vi "AviTrack2v2points(13_05_24).vi"() -> ()   [LabVIEW 2015]
uses:
  <vilib>/vision/Image Controls.llb/IMAQ Image.ctl
  <vilib>/vision/NI_Vision_Development_Module.lvlib
  <vilib>/ptbypt/NI_PtbyPt.lvlib
panel:
  out "Number of Matches (Color Location 2)":i32
  out "Number of Matches (Color Location 1)":i32
  out "substring":string
  in  "Enable":bool
  out "x+1":i32
  out "decimal integer string":string
  out "error out 2":errorcluster caption="error out"
  out "Saving Data":bool
  in  "error in (no error)":errorcluster
  out "Tiempo 2":dbl
  out "Tiempo":dbl
  out "Waveform Chart":dbl[](graph)
  out "Threshold":T1(plugin-control)
  out "Global Rectangle":dbl[](array[numeric])
  out "1°":i32
  out "2°":i32
  out "Dif. Puntos":i32
  in  "x = Centimetros reales":i32=20
  out "Dif. CM":dbl
  out "Waveform Chart 3":dbl(graph)
  out "Dist. CM":sgl
  out "Dist. Pixel":sgl
  out "IMA 3":T1(plugin-control)
  in  "Blue or Luminance":cluster{i32, i32}(slide)={0, 191} scale=0.0..255.0
  in  "Green or Saturation":cluster{i32, i32}(slide)={40, 231} scale=0.0..255.0
  in  "Red or Hue":cluster{i32, i32}(slide)={86, 222} scale=0.0..255.0
  out "Bounding Box[0].x":sgl
  out "error out":errorcluster
  out "Progress Bar 2":i32(slide) max=25 scale=-1.0..162.0
  in  "base path 2":path
  in  "Color Mode":u16(ring)=1 items=["RGB", "HSL", "HSV", "HSI"]
  out "Image":T1(plugin-control)
  in  "stop":bool
  out "Image Dst Out":T1
  out "Image 2":T1(plugin-control)
  in  "invert":bool
  out "IMA 2":T1(plugin-control)
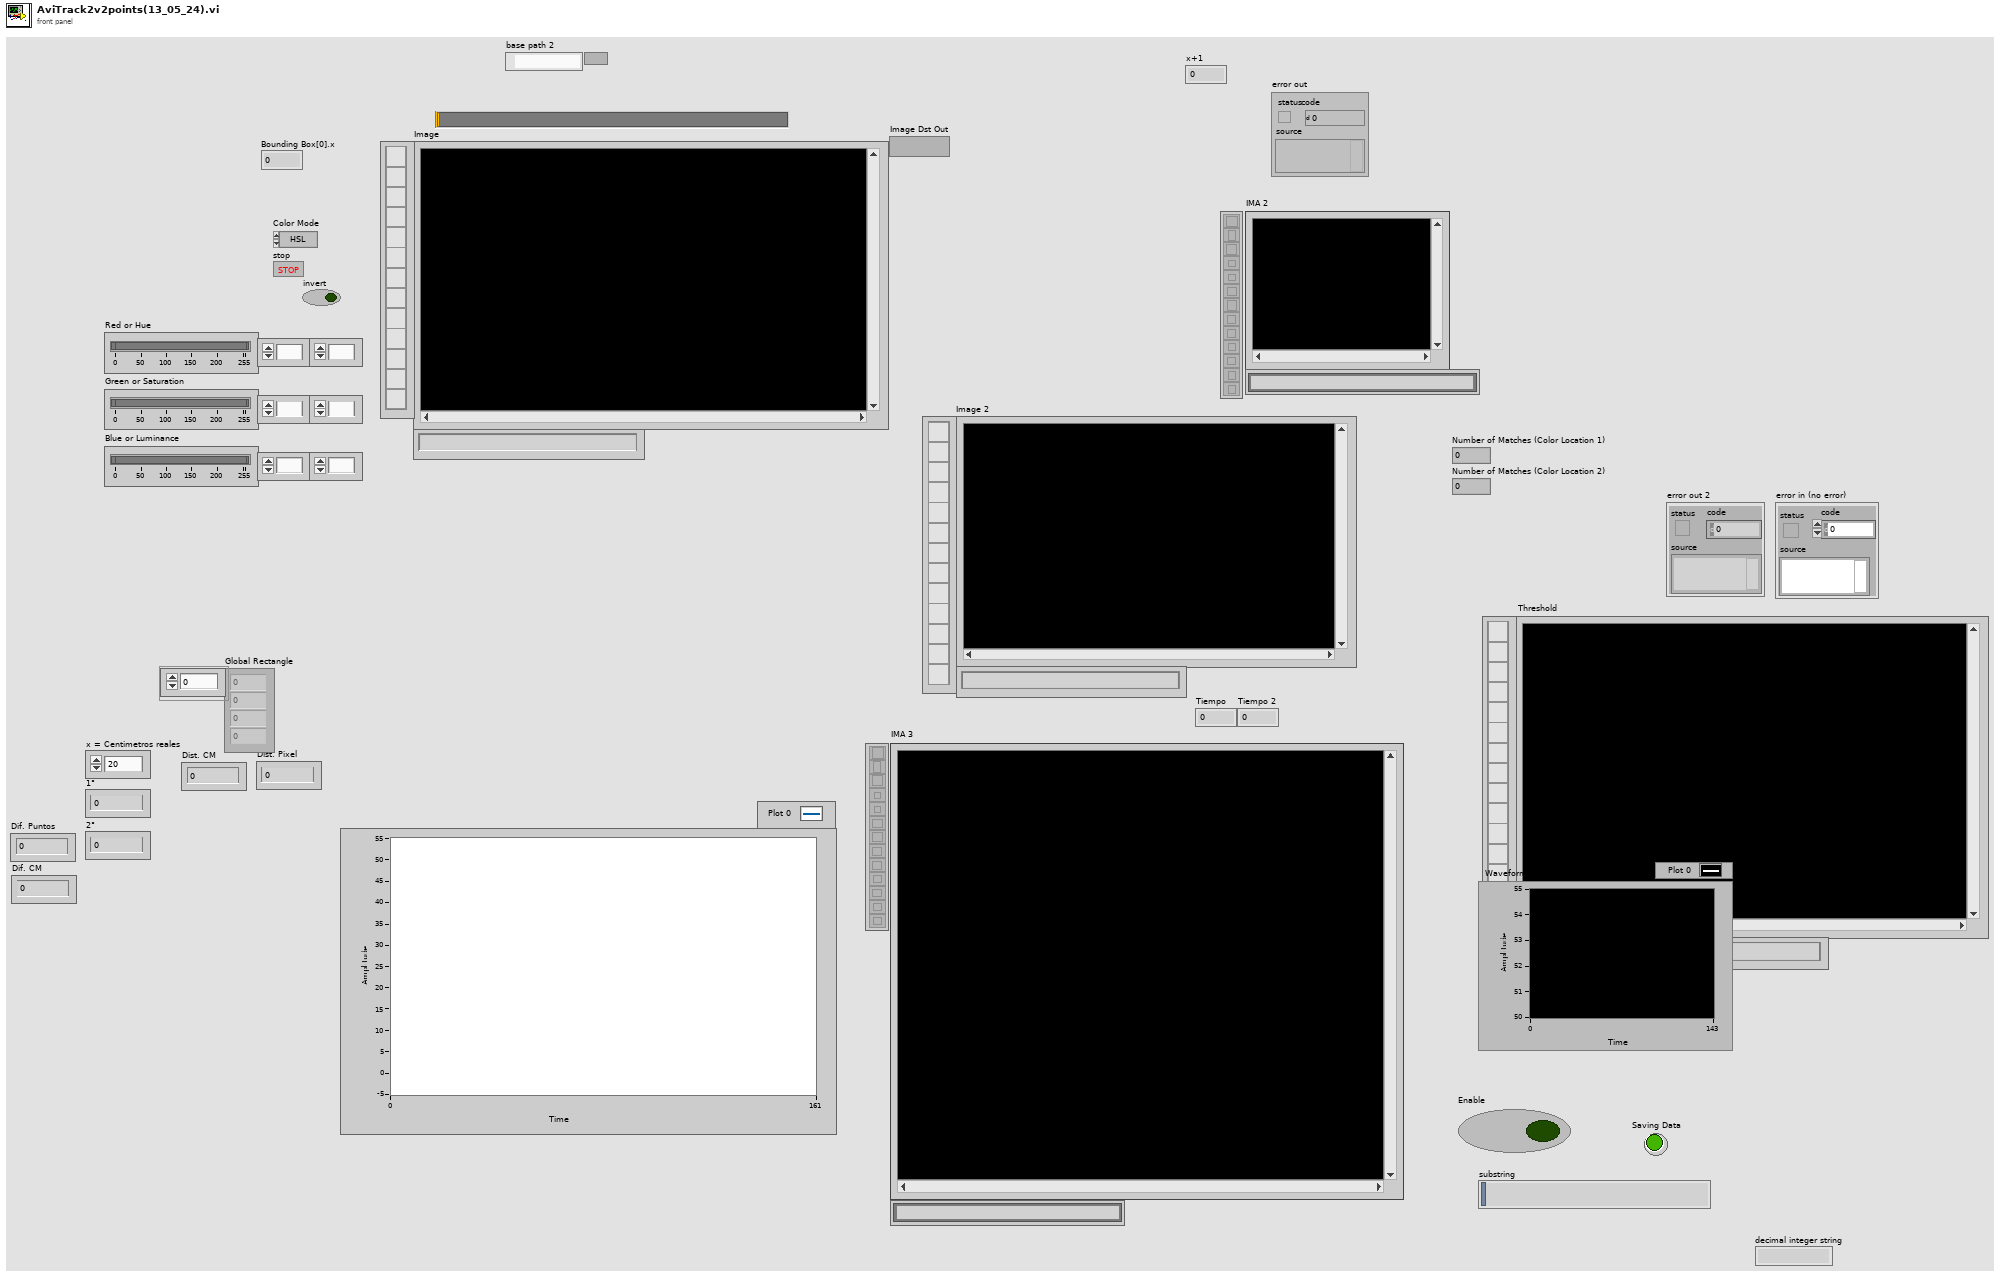
[diagram p1: front panel]
types:
  T1 = typedef "IMAQ Image.ctl" = refnum<image>
  T2 = typedef "Image Type" = u32
  T3 = typedef "IMAQ AVI2 Refnum.ctl" = refnum<k20>
  T4 = cluster{"Width":u32, "Height":u32, "Frames Per Second":u32, "Codec":string, "Has Data":bool}
  T5 = cluster{"Global Rectangle":i32[], "Contours":cluster{"Contour Type":u32, "ROI Type":u32, "Points":i32[]}[]}
  T6 = cluster{"Position":cluster{"x":sgl, "y":sgl}, "Angle":sgl, "Scale":sgl, "Score":sgl, "Bounding Box":cluster{"x":sgl, "y":sgl}[]}[]
  T7 = cluster{"Position":cluster{"x":sgl, "y":sgl}, "Angle":sgl, "Scale":sgl, "Score":sgl, "Bounding Box":cluster{"x":sgl, "y":sgl}[]}
  T8 = cluster{"Matches (Color Location 1)[0]":cluster{"Position":cluster{"x":sgl, "y":sgl}, "Angle":sgl, "Scale":sgl, "Score":sgl, "Bounding Box":cluster{"x":sgl, "y":sgl}[]}, "Matches (Color Location 1)[1]":cluster{"Position":cluster{"x":sgl, "y":sgl}, "Angle":sgl, "Scale":sgl, "Score":sgl, "Bounding Box":cluster{"x":sgl, "y":sgl}[]}, "Matches (Color Location 1)[2]":cluster{"Position":cluster{"x":sgl, "y":sgl}, "Angle":sgl, "Scale":sgl, "Score":sgl, "Bounding Box":cluster{"x":sgl, "y":sgl}[]}, "Matches (Color Location 1)[3]":cluster{"Position":cluster{"x":sgl, "y":sgl}, "Angle":sgl, "Scale":sgl, "Score":sgl, "Bounding Box":cluster{"x":sgl, "y":sgl}[]}}
  T9 = cluster{"Matches (Color Location 2)[0]":cluster{"Position":cluster{"x":sgl, "y":sgl}, "Angle":sgl, "Scale":sgl, "Score":sgl, "Bounding Box":cluster{"x":sgl, "y":sgl}[]}, "Matches (Color Location 2)[1]":cluster{"Position":cluster{"x":sgl, "y":sgl}, "Angle":sgl, "Scale":sgl, "Score":sgl, "Bounding Box":cluster{"x":sgl, "y":sgl}[]}, "Matches (Color Location 2)[2]":cluster{"Position":cluster{"x":sgl, "y":sgl}, "Angle":sgl, "Scale":sgl, "Score":sgl, "Bounding Box":cluster{"x":sgl, "y":sgl}[]}, "Matches (Color Location 2)[3]":cluster{"Position":cluster{"x":sgl, "y":sgl}, "Angle":sgl, "Scale":sgl, "Score":sgl, "Bounding Box":cluster{"x":sgl, "y":sgl}[]}}
  T10 = cluster{"Bounding Box[0]":cluster{"x":sgl, "y":sgl}, "Bounding Box[1]":cluster{"x":sgl, "y":sgl}, "Bounding Box[2]":cluster{"x":sgl, "y":sgl}, "Bounding Box[3]":cluster{"x":sgl, "y":sgl}}
  T11 = cluster{"[0]":sgl, "[1]":sgl, "[2]":sgl, "[3]":sgl}
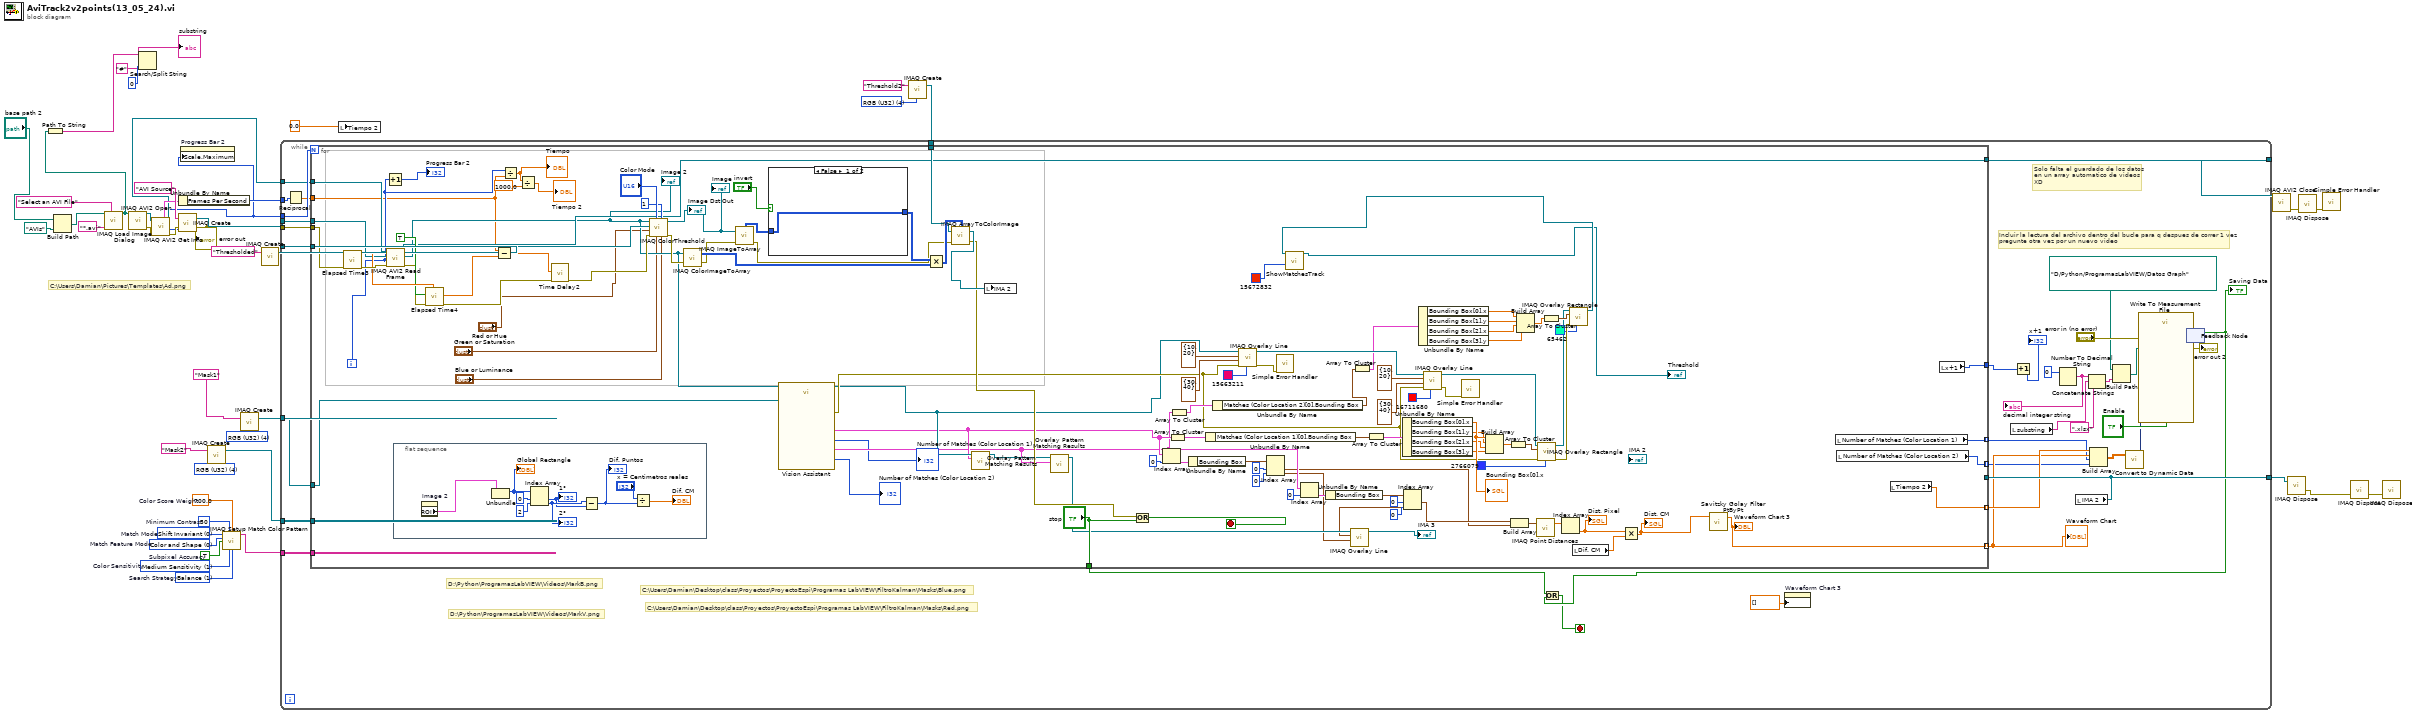
[diagram p0: block diagram]
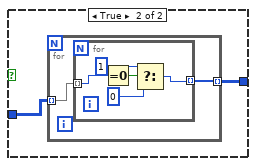
[diagram p2: hidden frame]
diagram:
  w13 = T2 4 items=["Grayscale (U8)", "Grayscale (I16)", "Grayscale (SGL)", "Complex (CSG)", "RGB (U32)", "HSL (U32)", "RGB (U64)", "Grayscale (U16)"] ("Image Type")
  w37 = T2 4 items=["Grayscale (U8)", "Grayscale (I16)", "Grayscale (SGL)", "Complex (CSG)", "RGB (U32)", "HSL (U32)", "RGB (U64)", "Grayscale (U16)"] ("Image Type")
  w39 = T2 4 items=["Grayscale (U8)", "Grayscale (I16)", "Grayscale (SGL)", "Complex (CSG)", "RGB (U32)", "HSL (U32)", "RGB (U64)", "Grayscale (U16)"] ("Image Type")
  w45 = TRUE  # Subpixel Accuracy
  w47 = u32 0 items=["Color and Shape", "Color", "Shape"]  # Match Feature Mode
  w41 = u32 1 items=["Conservative", "Balance", "Aggressive", "Very Aggressive"]  # Search Strategy
  w43 = 50  # Minimum Contrast
  w44 = sgl 700.0  # Color Score Weight
  w42 = u32 1 items=["Low Sensitivity", "Medium Sensitivity", "High Sensitivity"]  # Color Sensitivity
  w46 = u32 0 items=["Shift Invariant", "Rotation Invariant"]  # Match Mode
  # "C:\\Users\\Damian\\Pictures\\Templates\\Ad.png"
  n1 = Build Path(base path="base path 2", name or relative path=path "AVIs") -> (appended path=w6:path)
  n2 = call "IMAQ Load Image Dialog"("Prompt"="Select an AVI File" ("prompt"), "Pattern"="*.avi", "Start Path"=w6) -> ("Path"=w5:path)  [unwired: 6 in, 2 out]
  n3 = Path To String(path=w5) -> (string=w4:string)
  n4 = call "IMAQ AVI2 Open"("AVI File Path"=w5) -> ("error out"=w24:errorcluster, "AVI Refnum"=w23:T3)  [unwired: 2 in, 7 out]
  n5 = Search/Split String(string=w4, search string/char (-)="#", offset (0)=0) -> (match + rest of string=→"substring":string)  [unwired: 2 out]
  n6 = call "IMAQ AVI2 Get Info"("error in (no error)"=w24, "AVI Refnum"=w23) -> ("error out"=w22:errorcluster, "Image Type"=w21:T2, "Number of Frames"=w9:u32, "AVI Refnum (duplicate)"=w15:T3, "Frame Data"=w25:T4)  [unwired: 5 out]
  n7 = Unbundle By Name(w25) -> ("Frames Per Second"=w14:u32)
  n8 = call "IMAQ Create"("Image Name"="AVI Source", "Image Type"=w21, "error in (no error)"=w22) -> ("New Image"=w17:T1, "error out"=w16:errorcluster)  [unwired: 1 in, 1 out]
  "error out" <- w16
  n9 = property on="Progress Bar 2" class="Slide (strict)"("Scale.Maximum"=w9) -> ()  [unwired: 2 in, 2 out]
  n10 = call "IMAQ Create"("Image Name"="Mask2", "Image Type"=w37) -> ("New Image"=w33:T1)  [unwired: 3 in, 1 out]
  n11 = call "IMAQ Setup Match Color Pattern"("Match Mode"=w46, "Minimum Contrast"=w43, "Color Score Weight"=w44, "Match Feature Mode"=w47, "Subpixel Accuracy"=w45, "Color Sensitivity"=w42, "Search Strategy"=w41) -> ("Match Color Pattern Setup Data"=w32:string)  [unwired: 7 in, 1 out]
  n12 = call "IMAQ Create"("Image Name"="Mask1", "Image Type"=w39) -> ("New Image"=w34:T1)  [unwired: 3 in, 1 out]
  n13 = call "IMAQ Create"("Image Name"="Thresholded") -> ("New Image"=w35:T1)  [unwired: 3 in, 2 out]
  n14 = local write "Tiempo 2"(0.0 ("Tiempo 3")) -> ()
  n15 = call "IMAQ Create"("Image Name"="Threshold2", "Image Type"=w13) -> ("New Image"=w11:T1)  [unwired: 2 in, 2 out]
  n16 = while {
    tunnel: w34 -> [w83]
    tunnel: w33 -> [w82]
    tunnel: w32 -> [w81]
    tunnel: w35 -> [w80]
    tunnel: [w70] -> w29
    tunnel: w17 -> [w79]
    tunnel: w16 -> [w78]
    tunnel: w15 -> [w72]
    tunnel: w9 -> [w77]
    tunnel: w14 -> [w76]
    tunnel: w11 -> [w74]
    tunnel: [w73] -> w10
    stop <- w54 stop-if-true
    # "Incluir la lectura del archivo dentro del bucle para q despues de correr 1 vez\npregunte otra vez por un nuevo video"
    # "Solo falta el guardado de los datos \nen un array automatico de videos\nXD"
    # "D:\\Python\\ProgramasLabVIEW\\Videos\\MarkV.png"
    # "D:\\Python\\ProgramasLabVIEW\\Videos\\MarkB.png"
    # "C:\\Users\\Damian\\Desktop\\class\\Proyectos\\ProyectoEspi\\Programas LabVIEW\\FiltroKalman\\Masks\\Red.png"
    # "C:\\Users\\Damian\\Desktop\\class\\Proyectos\\ProyectoEspi\\Programas LabVIEW\\FiltroKalman\\Masks\\Blue.png"
    n17 = Reciprocal(x=w76) -> (1/x=w75:dbl)
    n18 = property on="Waveform Chart 3" class="WFChart (strict)"("History Data"=dbl[] []) -> ()  [unwired: 2 in, 2 out]
    n19 = local read "substring"() -> (w53:string)
    n20 = Number To Decimal String(number=0) -> (decimal integer string=w66:string)  [unwired: 1 in]
    "decimal integer string" <- w66
    n21 = local read "IMA 2"() -> (w70:T1)
    n22 = for {
      N: w77 -> [_]
      tunnel: w83 -> [w161]
      tunnel: w82 -> [_]
      tunnel: w81 -> [_]
      tunnel: w80 -> [w183]
      tunnel: w70 -> [_]
      tunnel: w79 -> [w163]
      tunnel: w78 -> [w174]
      tunnel: w75 -> [w93]
      tunnel: ["stop"] -> w56
      tunnel: w74 -> [w168]
      tunnel: [w165] -> w73
      tunnel: w72 -> [w164]
      tunnel: [w96] -> w62 mode=indexing
      tunnel: [w89] -> w63 mode=indexing
      tunnel: [w88] -> w60
      tunnel: [w85] -> w51 mode=indexing
      tunnel: [w84] -> w50 mode=indexing
      i -> [w94]
      stop <- w169 stop-if-true
      n23 = call "Elapsed Time3"("error in (no error)"=w174) -> ("Present (s)"=w180:dbl, "error out"=w181:errorcluster)  [unwired: 11 in, 6 out]
      n24 = Increment(x=w94) -> (x+1=→"Progress Bar 2":i32)
      n25 = call "IMAQ AVI2 Read Frame"("error in (no error)"=w181, "Frame Number"=w94, "Image"=w163, "AVI Refnum"=w164) -> ("error out"=w178:errorcluster, "Image Out"=w162:T1, "AVI Refnum (duplicate)"=w165:T3)  [unwired: 5 out]
      "Image 2" <- w162
      n26 = flat-sequence {
        frame #0 {
          n27 = property on="Image 2" class="ImageControl"() -> ("ROI"=w192:T5)  [unwired: 2 in, 2 out]
          n28 = Unbundle(w192) -> ("Global Rectangle"=w200:i32[])  [unwired: 1 out]
          "Global Rectangle" <- w200
          n29 = Index Array(array=w200, index #1=0 ("index"), index #2=2 ("index")) -> (element #1=w196:i32, element #2=w197:i32)
          "1°" <- w196
          "2°" <- w197
          n30 = Subtract(x=w197, y=w196) -> (x-y=w195:i32)
          "Dif. Puntos" <- w195
          n31 = Divide(x="x = Centimetros reales", y=w195) -> (x/y=→"Dif. CM":dbl)
        }
      }
      n32 = call "Elapsed Time4"("Reset"=TRUE, "error in (no error)"=w178, "Set Start Time (s)"=w180) -> ("Elapsed Time (s)"=w177:dbl, "error out"=w176:errorcluster)  [unwired: 9 in, 6 out]
      n33 = Subtract(x=w93, y=w177) -> (x-y=w95:dbl)
      n34 = Divide(x=w94, y=w93) -> (x/y=w92:dbl)
      "Tiempo" <- w92
      n35 = Divide(x=w92, y=1000.0) -> (x/y=→"Tiempo 2":dbl)
      n36 = call "Time Delay2"("error in (no error)"=w176, "Delay Time (s)"=w95) -> ("error out"=w173:errorcluster)  [unwired: 9 in]
      n37 = call "IMAQ ColorThreshold"("Blue or Luma or Val or Inten Range"="Blue or Luminance", "Replace Value"=1, "Green or Sat Range"="Green or Saturation", "Color Mode"="Color Mode", "error in (no error)"=w173, "Red or Hue Range"="Red or Hue", "Image Dst"=w183, "Image Src"=w162) -> ("error out"=w172:errorcluster, "Image Dst Out"=w189:T1)  [unwired: 2 in]
      "Image" <- w189
      "Image Dst Out" <- w189
      n38 = call "IMAQ ColorImageToArray"("Image"=w162, "error in (no error)"=w172) -> ("Image Pixels (U32)"=w186:u32[][], "error out"=w171:errorcluster)  [unwired: 2 in, 1 out]
      n39 = call "IMAQ ImageToArray"("error in (no error)"=w171, "Image"=w189) -> ("error out"=w167:errorcluster, "Image Pixels (U8)"=w184:u8[][])  [unwired: 2 in, 3 out]
      n40 = case shown="False" "invert" {
        tunnel: w184 -> [w201 w203]
        tunnel: [w201 w202] -> w187
        frame False {
        }
        frame True {
          n41 = for {
            tunnel: w203 -> [w205] mode=indexing
            tunnel: [w204] -> w202 mode=indexing
            n42 = for {
              tunnel: w205 -> [w206] mode=indexing
              tunnel: [w207] -> w204 mode=indexing
              n43 = Equal To 0?(x=w206) -> (x = 0?=w210:bool)
              n44 = Select(t=1, s=w210, f=0) -> (s? t:f=w207:i32)
            }
          }
        }
      }
      n45 = call "Vision Assistant"("Image In"=w162, "Image Dst"=w161) -> ("Image Out"=w122:T1, "Matches (Color Location 1)"=w114:T6, "Matches (Color Location 2)"=w108:T6, "Number of Matches (Color Location 1)"=→"Number of Matches (Color Location 1)":i32, "Number of Matches (Color Location 2)"=→"Number of Matches (Color Location 2)":i32, "error out"=w126:errorcluster)  [unwired: 20 in]
      n46 = Multiply(x=w187, y=w186) -> (x*y=w185:u32[][])
      n47 = call "IMAQ ArrayToColorImage"("Image Pixels (U32)"=w185, "Image"=w168, "error in (no error)"=w167) -> ("Image Out"=w182:T1, "error out"=w166:errorcluster)  [unwired: 2 in]
      n48 = call "Overlay Pattern Matching Results.vi"("Matches"=w114, "Image"=w122) -> ("Image Out"=w121:T1)  [unwired: 8 in, 1 out]
      n49 = local write "IMA 2"(w182) -> ()
      n50 = call "Overlay Pattern Matching Results.vi"("Matches"=w108, "Image"=w121) -> ("Image Out"=w120:T1)  [unwired: 8 in, 1 out]
      n51 = Or(x=w166, y="stop") -> (x .or. y?=w169:bool)
      n52 = Index Array(array=w114, index=0) -> (element=w118:T7)
      n53 = Array To Cluster(array=w114) -> (cluster=w142:T8)
      n54 = Array To Cluster(array=w108) -> (cluster=w141:T9)
      n55 = Unbundle By Name(w118) -> ("Bounding Box"=w117:cluster{"x":sgl, "y":sgl}[])
      n56 = Unbundle By Name(w142) -> ("Matches (Color Location 1)[0].Bounding Box"=w160:cluster{"x":sgl, "y":sgl}[])
      n57 = Unbundle By Name(w141) -> ("Matches (Color Location 2)[0].Bounding Box"=w140:cluster{"x":sgl, "y":sgl}[])
      n58 = call "IMAQ Overlay Line"("Color"=u32 15663211, "error in (no error)"=w126, "End Point"=cluster{"X":i32, "Y":i32} {"X"=30, "Y"=40} ("Start Point"), "Start Point"=cluster{"X":i32, "Y":i32} {"X"=10, "Y"=20}, "Image"=w122) -> ("error out"=w144:errorcluster, "Image Out"=w151:T1)  [unwired: 5 in]
      n59 = Index Array(array=w117, index #1=0 ("index"), index #2=0 ("index")) -> (element #1=w100:cluster{"x":sgl, "y":sgl}, element #2=w107:cluster{"x":sgl, "y":sgl})
      n60 = call <vilib>:"Simple Error Handler.vi"("error in (no error)"=w144) -> ()  [unwired: 4 in, 5 out]
      n61 = Index Array(array=w108, index=0) -> (element=w112:T7)
      n62 = Unbundle By Name(w112) -> ("Bounding Box"=w111:cluster{"x":sgl, "y":sgl}[])
      n63 = Array To Cluster(array=w140) -> (cluster=w139:T10)
      n64 = Array To Cluster(array=w160) -> (cluster=w159:T10)
      n65 = Unbundle By Name(w159) -> ("Bounding Box[0].x"=w158:sgl, "Bounding Box[1].y"=w155:sgl, "Bounding Box[2].x"=w156:sgl, "Bounding Box[3].y"=w157:sgl)
      "Bounding Box[0].x" <- w158
      n66 = Index Array(array=w111, index #1=0 ("index"), index #2=0 ("index")) -> (element #1=w101:cluster{"x":sgl, "y":sgl}, element #2=w106:cluster{"x":sgl, "y":sgl})
      n67 = call "IMAQ Overlay Line"("End Point"=w107, "Start Point"=w106, "Image"=w120) -> ("Image Out"=→"IMA 3":T1)  [unwired: 7 in, 1 out]
      n68 = Unbundle By Name(w139) -> ("Bounding Box[0].x"=w138:sgl, "Bounding Box[1].y"=w137:sgl, "Bounding Box[2].x"=w136:sgl, "Bounding Box[3].y"=w135:sgl)
      n69 = call "IMAQ Overlay Line"("Color"=u32 16711680, "error in (no error)"=w126, "End Point"=cluster{"X":i32, "Y":i32} {"X"=30, "Y"=40} ("Start Point"), "Start Point"=cluster{"X":i32, "Y":i32} {"X"=10, "Y"=20}, "Image"=w151) -> ("error out"=w143:errorcluster, "Image Out"=w152:T1)  [unwired: 5 in]
      n70 = call <vilib>:"Simple Error Handler.vi"("error in (no error)"=w143) -> ()  [unwired: 4 in, 5 out]
      n71 = Build Array(w158, w155, w156, w157) -> (w154:sgl[])
      n72 = Array To Cluster(array=w154) -> (cluster=w153:T11)
      n73 = Build Array(w101, w100) -> (w104:cluster{"x":sgl, "y":sgl}[])
      n74 = Build Array(w138, w137, w136, w135) -> (w134:sgl[])
      n75 = call "IMAQ Point Distances"("Points"=w104) -> ("Distances"=w103:sgl[])  [unwired: 4 in, 1 out]
      n76 = call "IMAQ Overlay Rectangle"("Color"=u32 2766079, "error in (no error)"=w126, "Rectangle"=w153, "Image"=w152) -> ("error out"=w131:errorcluster, "Image Out"=w132:T1)  [unwired: 6 in]
      n77 = Array To Cluster(array=w134) -> (cluster=w133:T11)
      n78 = Index Array(array=w103) -> (element=w102:sgl)  [unwired: 1 in]
      "Dist. Pixel" <- w102
      n79 = call "IMAQ Overlay Rectangle"("Color"=u32 65462, "error in (no error)"=w131, "Rectangle"=w133, "Image"=w132) -> ("Image Out"=w128:T1)  [unwired: 6 in, 1 out]
      n80 = call "ShowMatchesTrack.vi"("Refnum in"=w128, "Color"=u32 15672832) -> ("Refnum out"=→"Threshold":T1)  [unwired: 8 in, 5 out]
      n81 = local read "Dif. CM"() -> (w98:dbl)
      n82 = Multiply(x=w102, y=w98) -> (x*y=w99:dbl)
      "Dist. CM" <- w99
      n83 = call <vilib>:"Savitzky Golay Filter PtByPt.vi"("x"=w99) -> ("Filtered x"=w96:dbl)  [unwired: 3 in, 1 out]
      "Waveform Chart 3" <- w96
      n84 = local read "Number of Matches (Color Location 1)"() -> (w85:i32)
      n85 = local read "Number of Matches (Color Location 2)"() -> (w84:i32)
      n86 = local read "Tiempo 2"() -> (w89:dbl)
      n87 = local read "x+1"() -> (w88:i32)
    }
    "Waveform Chart" <- w62
    n88 = Increment(x=w60) -> (x+1=→"x+1":i32)
    n89 = Concatenate Strings(w66, w53, ".xlsx" ("string")) -> (w65:string)
    n90 = Build Array(w63, w62, w51, w50) -> (w49:dbl[][])
    n91 = Build Path(base path=path "D:/Python/ProgramasLabVIEW/Datos Graph", name or relative path=w65) -> (appended path=w64:path)
    n92 = call "Convert to Dynamic Data"("2D Array"=w49) -> ("Dynamic Data Type"=w48:dynamicdata)  [unwired: 3 in]
    n93 = call "Write To Measurement File"("Signals"=w48, "Enable"="Enable", "error in (no error)"="error in (no error)", "Filename"=w64) -> ("Saving Data"=w57:bool, "error out"=→"error out 2":errorcluster)  [unwired: 13 in, 1 out]
    n94 = feedback-in #1(w57) -> ()
    n95 = feedback #1() -> (w55:bool)  [unwired: 1 in]
    "Saving Data" <- w55
    n96 = Or(x=w56, y=w55) -> (x .or. y?=w54:bool)
  }
  n97 = call "IMAQ AVI2 Close"("AVI Refnum"=w10) -> ("error out"=w27:errorcluster)  [unwired: 1 in, 9 out]
  n98 = call "IMAQ Dispose"("Image"=w29) -> ("error out"=w30:errorcluster)  [unwired: 5 in]
  n99 = call "IMAQ Dispose"("error in (no error)"=w27) -> ("error out"=w28:errorcluster)  [unwired: 2 in, 3 out]
  n100 = call <vilib>:"Simple Error Handler.vi"("error in (no error)"=w28) -> ()  [unwired: 1 in, 8 out]
  n101 = call "IMAQ Dispose"("error in (no error)"=w30) -> ("error out"=w31:errorcluster)  [unwired: 5 in]
  n102 = call "IMAQ Dispose"("error in (no error)"=w31) -> ()  [unwired: 5 in, 1 out]
